vi "AlliGator Load Local IRFs.vi"(8 "error in (no error)":errorcluster, 11 "File Path":path) -> (0 "error out":errorcluster, 1 "Message":string, 2 "IRF Array Time Axis":dbl[](array[numeric]), 3 "[[IRFs]]":dbl[][](array[numeric]), 4 "# IRFs":i32, 5 "Dataset Information v1":T1)   [LabVIEW 2021, in "AlliGator IRF.lvlib"]
uses:
  AlliGator IRF.lvlib
  Files/AlliGator FLI Dataset Information v1.ctl
  <vilib>/addons/h5labview2/file/H5Fmode.ctl
  AlliGator Local IRFs HDF5 File Sections.ctl
  <vilib>/Utility/error.llb/Error Cluster From Error Code.vi
  <vilib>/addons/h5labview2/base/lib_path.vi
  <vilib>/addons/h5labview2/base/H5Equery.vi
  <vilib>/ErrorRing/Error Ring.xnode
  <vilib>/addons/h5labview2/dataset/H5Dread.llb/H5Dread.xnode
  <vilib>/addons/h5labview2/file/H5F.lvlib
  <vilib>/addons/h5labview2/group/H5G.lvlib
  Variant/Variant.lvlib
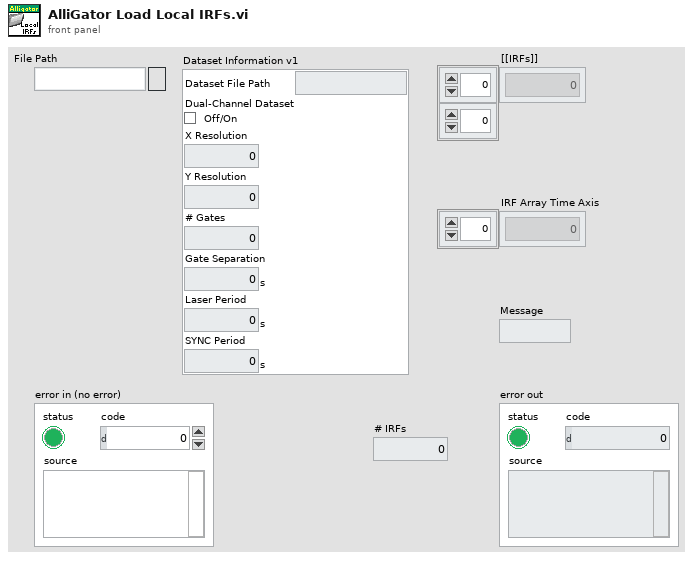
[diagram p1: front panel]
types:
  T1 = typedef "AlliGator IRF.lvlib/AlliGator FLI Dataset Information v1.ctl" = cluster{"Dataset File Path":path, "Dual-Channel Dataset":bool, "X Resolution":i32, "Y Resolution":i32, "# Gates":i32, "Gate Separation":dbl[unit], "Laser Period":dbl[unit], "SYNC Period":dbl[unit]}
  T2 = typedef "AlliGator IRF.lvlib/AlliGator Local IRFs HDF5 File Sections.ctl" = enum16{"File Information", "Dataset Information", "Local IRFs Data"}
  T3 = typedef "H5F.lvlib/H5Fmode.ctl" = enum16{"read-only", "read-write", "overwrite", "create new", "open or create"}
  T4 = typedef "hid_t.ctl" = i64
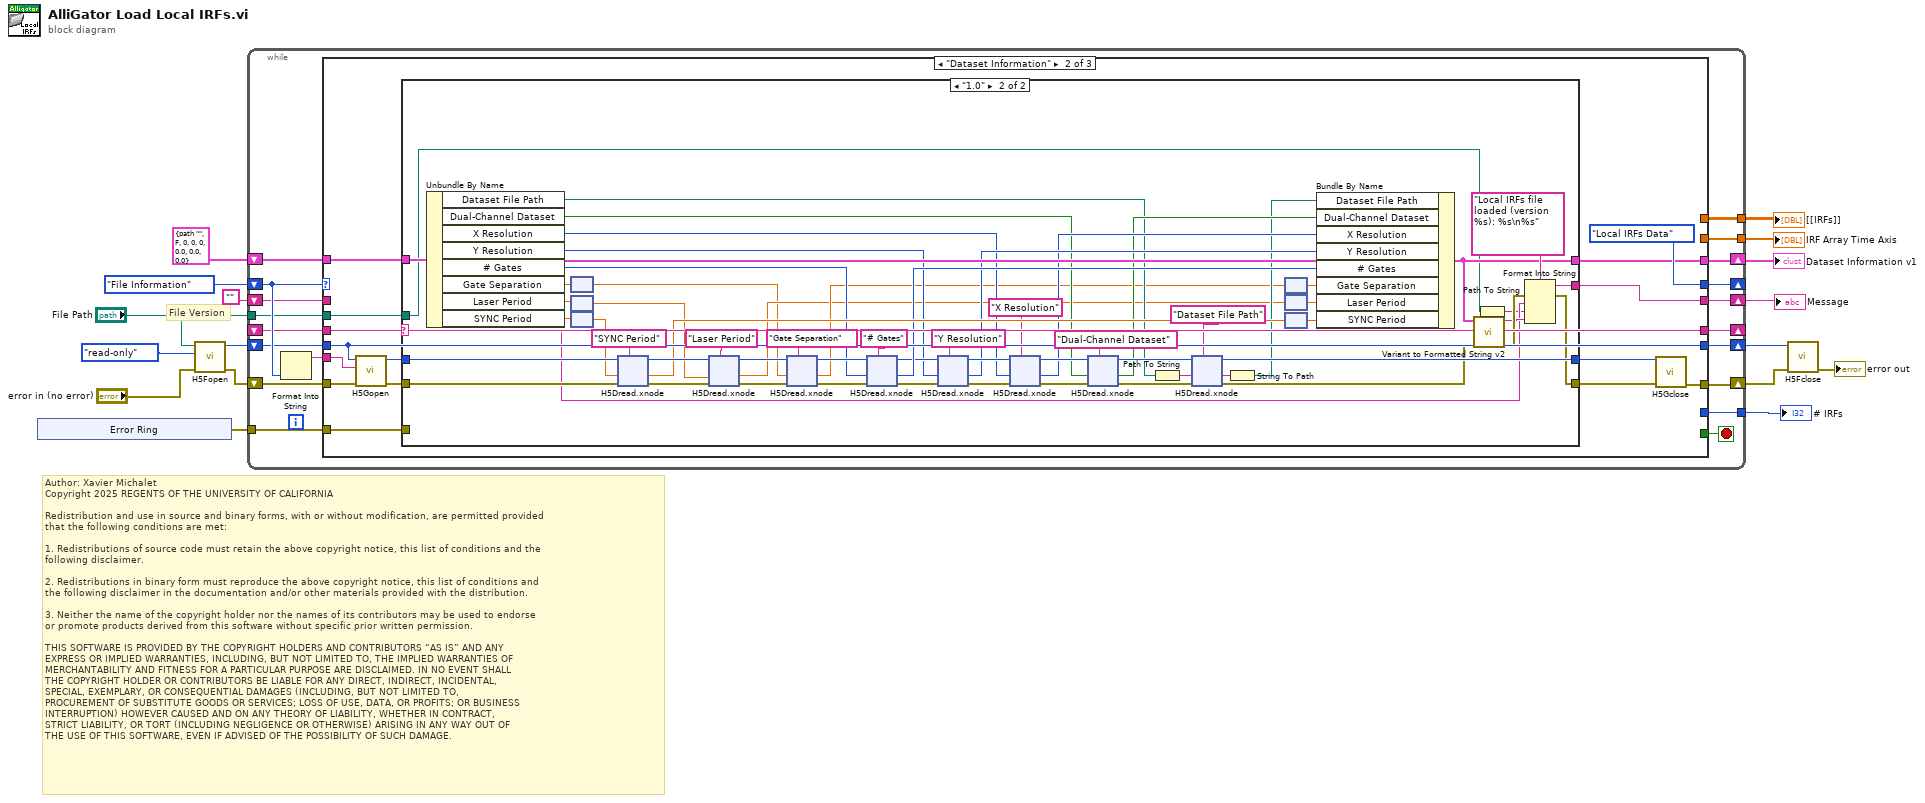
[diagram p0: block diagram]
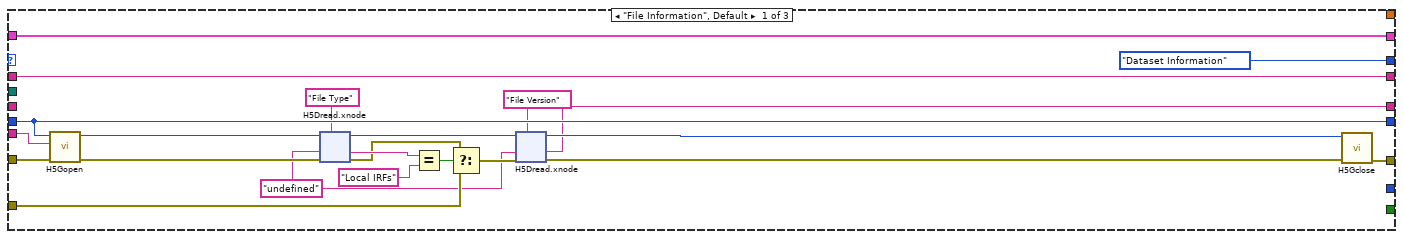
[diagram p2: hidden frame]
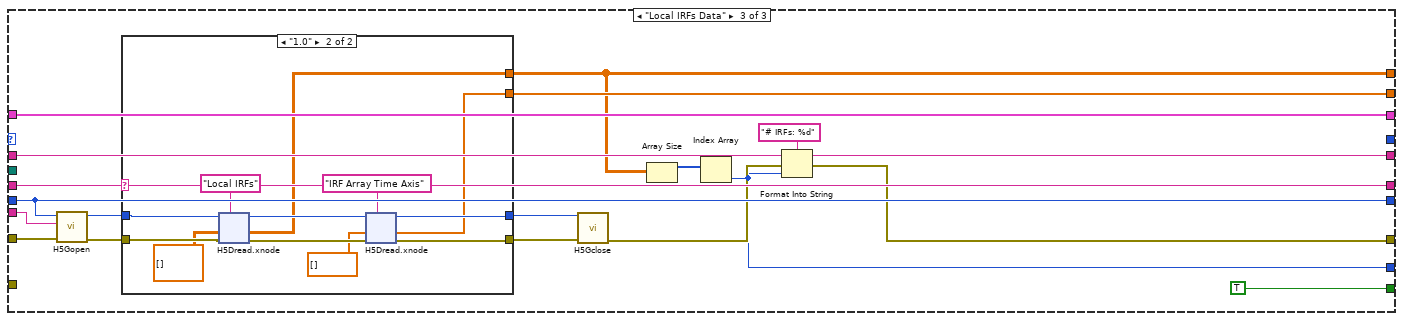
[diagram p4: hidden frame]
diagram:
  # "Author: Xavier Michalet\nCopyright 2025 REGENTS OF THE UNIVERSITY OF CALIFORNIA\n\nRedistribution and use in source and binary forms, with or without modification, are permitted provided\nthat the following conditions are met:\n\n1. Redistributions of source code must retain the above copyright notice, this list of conditions and the\nfollowing disclaimer.\n\n2. Redistributions in binary form must reproduce the above copyright notice, this list of conditions and\nthe following disclaimer in the documentation and/or other materials provided with the distribution.\n\n3. Neither the name of the copyright holder nor the names of its contributors may be used to endorse \nor promote products derived from this software without specific prior written permission.\n\nTHIS SOFTWARE IS PROVIDED BY THE COPYRIGHT HOLDERS AND CONTRIBUTORS “AS IS” AND ANY \nEXPRESS OR IMPLIED WARRANTIES, INCLUDING, BUT NOT LIMITED TO, THE IMPLIED WARRANTIES OF\nMERCHANTABILITY AND FITNESS FOR A PARTICULAR PURPOSE ARE DISCLAIMED. IN NO EVENT SHALL\nTHE COPYRIGHT HOLDER OR CONTRIBUTORS BE LIABLE FOR ANY DIRECT, INDIRECT, INCIDENTAL, \nSPECIAL, EXEMPLARY, OR CONSEQUENTIAL DAMAGES (INCLUDING, BUT NOT LIMITED TO, \nPROCUREMENT OF SUBSTITUTE GOODS OR SERVICES; LOSS OF USE, DATA, OR PROFITS; OR BUSINESS\nINTERRUPTION) HOWEVER CAUSED AND ON ANY THEORY OF LIABILITY, WHETHER IN CONTRACT, \nSTRICT LIABILITY, OR TORT (INCLUDING NEGLIGENCE OR OTHERWISE) ARISING IN ANY WAY OUT OF\nTHE USE OF THIS SOFTWARE, EVEN IF ADVISED OF THE POSSIBILITY OF SUCH DAMAGE."
  # "File Version"
  n1 = xnode "Error Ring"() -> ("error out"=w12:errorcluster)
  n2 = call <vilib>:"H5Fopen.vi"("error in (no error)"="error in (no error)", "mode (read-only)"=H5Fmode."read-only", "path"="File Path") -> ("error out"=w13:errorcluster, "ref out"=w14:T4)  [unwired: 7 in]
  n3 = while {
    shift-right: [w28] -> _
    shift-left: AlliGator_Local_IRFs_HDF5_File_Sections."File Information" -> [w36]
    shift-right: [w33] -> w9
    shift-left: w14 -> [w34]
    shift-right: [w31] -> w8
    shift-left: w13 -> [w32]
    tunnel: w12 -> [w30]
    shift-right: [w29] -> _
    shift-left: _ -> [w27]
    shift-right: [w24] -> w10
    shift-left: T1 {"Dataset File Path"=path "", "Dual-Channel Dataset"=FALSE, "X Resolution"=0, "Y Resolution"=0, "# Gates"=0, "Gate Separation"=0.0, "Laser Period"=0.0, "SYNC Period"=0.0} ("Dataset Information v1") -> [w26]
    shift-right: [w21] -> w4
    shift-left: "" -> [w20]
    tunnel: [w23] -> w7
    tunnel: [w22] -> w6
    tunnel: [w19] -> w3
    tunnel: "File Path" -> [w18]
    stop <- w25 stop-if-true
    n4 = Format Into String(w36) -> (resulting string=w35:string)  [unwired: 3 in, 1 out]
    n5 = case shown="\"Dataset Information\"" w36 {
      tunnel: w35 -> [w57 w102 w294]
      tunnel: w34 -> [w58 w103 w297]
      tunnel: [w58 w103 w297] -> w33
      tunnel: w32 -> [w56 w101 w304]
      tunnel: [w50 w96 w287] -> w31
      tunnel: w30 -> [w44 w95 _]
      tunnel: [w40 w94 w298] -> w29
      tunnel: [AlliGator_Local_IRFs_HDF5_File_Sections."Dataset Information" AlliGator_Local_IRFs_HDF5_File_Sections."Local IRFs Data" _] -> w28
      tunnel: w27 -> [_ w94 w298]
      tunnel: w26 -> [w38 w92 w295]
      tunnel: [_ _ TRUE] -> w25
      tunnel: [w38 w91 w295] -> w24
      tunnel: [_ _ w290] -> w23
      tunnel: [_ _ w296] -> w22
      tunnel: [w37 w90 w291] -> w21
      tunnel: w20 -> [w37 _ w292]
      tunnel: [_ _ w286] -> w19
      tunnel: w18 -> [_ w89 _]
      frame "File Information", Default {
        w42 = "undefined" ("name")
        n6 = call <vilib>:"H5Gopen.vi"("error in (no error)"=w56, "name"=w57, "ref in"=w58) -> ("error out"=w54:errorcluster, "group out"=w55:T4)  [unwired: 7 in]
        n7 = xnode "H5Dread.xnode"("dataset name (this)"="File Type" ("name"), "error in (no error)"=w54, "default"=w42, "ref in"=w55) -> ("error out"=w45:errorcluster, "data"=w48:string, "ref out"=w53:i64)  [unwired: 2 in, 1 out]
        n8 = Equal?(x=w48, y="Local IRFs" ("name")) -> (x = y?=w46:bool)
        n9 = Select(t=w45, s=w46, f=w44) -> (s? t:f=w43:errorcluster)
        n10 = xnode "H5Dread.xnode"("dataset name (this)"="File Version" ("dataset name"), "error in (no error)"=w43, "default"=w42, "ref in"=w53) -> ("error out"=w52:errorcluster, "data"=w40:string, "ref out"=w51:i64)  [unwired: 2 in, 1 out]
        n11 = call <vilib>:"H5Gclose.vi"("error in (no error)"=w52, "group in"=w51) -> ("error out"=w50:errorcluster)  [unwired: 9 in]
      }
      frame "Dataset Information" {
        n12 = call <vilib>:"H5Gopen.vi"("error in (no error)"=w101, "name"=w102, "ref in"=w103) -> ("error out"=w99:errorcluster, "group out"=w100:T4)  [unwired: 7 in]
        n13 = case shown="\"1.0\"" w94 {
          selector: w94 -> [_ w118]
          tunnel: w100 -> [w105 w165]
          tunnel: w99 -> [w104 w164]
          tunnel: [w104 w120] -> w98
          tunnel: [w105 w138] -> w97
          tunnel: w95 -> [_ _]
          tunnel: w92 -> [_ w159]
          tunnel: [_ w123] -> w91
          tunnel: [_ w124] -> w90
          tunnel: w89 -> [_ w107]
          frame "", Default {
          }
          frame "1.0" {
            n14 = Unbundle By Name(w159) -> ("Dataset File Path"=w129:path, "Dual-Channel Dataset"=w131:bool, "X Resolution"=w133:i32, "Y Resolution"=w146:i32, "# Gates"=w151:i32, "Gate Separation"=w111:dbl[unit], "Laser Period"=w110:dbl[unit], "SYNC Period"=w160:dbl[unit])
            n15 = node(w111) -> (w108:dbl)
            n16 = node(w110) -> (w109:dbl)
            n17 = node(w160) -> (w117:dbl)
            n18 = xnode "H5Dread.xnode"("dataset name (this)"="SYNC Period" ("name"), "error in (no error)"=w164, "default"=w117, "ref in"=w165) -> ("error out"=w157:errorcluster, "data"=w158:dbl, "ref out"=w163:i64)  [unwired: 2 in, 1 out]
            n19 = xnode "H5Dread.xnode"("dataset name (this)"="Laser Period" ("dataset name"), "error in (no error)"=w157, "default"=w109, "ref in"=w163) -> ("error out"=w155:errorcluster, "data"=w114:dbl, "ref out"=w156:i64)  [unwired: 2 in, 1 out]
            n20 = xnode "H5Dread.xnode"("dataset name (this)"="Gate Separation" ("dataset name"), "error in (no error)"=w155, "default"=w108, "ref in"=w156) -> ("error out"=w153:errorcluster, "data"=w115:dbl, "ref out"=w154:i64)  [unwired: 2 in, 1 out]
            n21 = xnode "H5Dread.xnode"("dataset name (this)"="# Gates" ("dataset name"), "error in (no error)"=w153, "default"=w151, "ref in"=w154) -> ("error out"=w148:errorcluster, "data"=w149:i32, "ref out"=w147:i64)  [unwired: 2 in, 1 out]
            n22 = xnode "H5Dread.xnode"("dataset name (this)"="Y Resolution" ("dataset name"), "error in (no error)"=w148, "default"=w146, "ref in"=w147) -> ("error out"=w142:errorcluster, "data"=w134:i32, "ref out"=w141:i64)  [unwired: 2 in, 1 out]
            n23 = xnode "H5Dread.xnode"("dataset name (this)"="X Resolution" ("dataset name"), "error in (no error)"=w142, "default"=w133, "ref in"=w141) -> ("error out"=w143:errorcluster, "data"=w132:i32, "ref out"=w140:i64)  [unwired: 2 in, 1 out]
            n24 = xnode "H5Dread.xnode"("dataset name (this)"="Dual-Channel Dataset" ("dataset name"), "error in (no error)"=w143, "default"=w131, "ref in"=w140) -> ("error out"=w144:errorcluster, "data"=w130:bool, "ref out"=w139:i64)  [unwired: 2 in, 1 out]
            n25 = Path To String(path=w129) -> (string=w128:string)
            n26 = xnode "H5Dread.xnode"("dataset name (this)"="Dataset File Path" ("dataset name"), "error in (no error)"=w144, "default"=w128, "ref in"=w139) -> ("error out"=w121:errorcluster, "data"=w125:string, "ref out"=w138:i64)  [unwired: 2 in, 1 out]
            n27 = String To Path(string=w125) -> (path=w127:path)
            n28 = node(w115) -> (w113:dbl[unit])
            n29 = node(w114) -> (w112:dbl[unit])
            n30 = node(w158) -> (w116:dbl[unit])
            n31 = Bundle By Name(cluster=w159, "Dataset File Path"=w127, "Dual-Channel Dataset"=w130, "X Resolution"=w132, "Y Resolution"=w134, "# Gates"=w149, "Gate Separation"=w113, "Laser Period"=w112, "SYNC Period"=w116) -> (w123:T1)
            n32 = call "Variant to Formatted String v2.vi"("error in (no error)"=w121, "Anything"=w123) -> ("error out"=w122:errorcluster, "String"=w119:string)  [unwired: 8 in]
            n33 = Path To String(path=w107) -> (string=w106:string)
            n34 = Format Into String(format string="Local IRFs file loaded (version %s): %s\n%s", error in=w122, w118, w106, w119) -> (resulting string=w124:string, error out=w120:errorcluster)  [unwired: 1 in]
          }
        }
        n35 = call <vilib>:"H5Gclose.vi"("error in (no error)"=w98, "group in"=w97) -> ("error out"=w96:errorcluster)  [unwired: 9 in]
      }
      frame "Local IRFs Data" {
        n36 = call <vilib>:"H5Gopen.vi"("error in (no error)"=w304, "name"=w294, "ref in"=w297) -> ("error out"=w303:errorcluster, "group out"=w302:T4)  [unwired: 7 in]
        n37 = case shown="\"1.0\"" w298 {
          tunnel: w303 -> [w306 w315]
          tunnel: w302 -> [w305 w314]
          tunnel: [w306 w311] -> w301
          tunnel: [w305 w312] -> w300
          tunnel: [_ w309] -> w290
          tunnel: [_ w307] -> w296
          frame "", Default {
          }
          frame "1.0" {
            n38 = xnode "H5Dread.xnode"("dataset name (this)"="Local IRFs" ("name"), "error in (no error)"=w315, "default"=dbl[][] [] ("[[IRFs]]"), "ref in"=w314) -> ("error out"=w318:errorcluster, "data"=w309:dbl[][], "ref out"=w313:i64)  [unwired: 2 in, 1 out]
            n39 = xnode "H5Dread.xnode"("dataset name (this)"="IRF Array Time Axis" ("dataset name"), "error in (no error)"=w318, "default"=dbl[] [] ("IRF Array Time Axis"), "ref in"=w313) -> ("error out"=w311:errorcluster, "data"=w307:dbl[], "ref out"=w312:i64)  [unwired: 2 in, 1 out]
          }
        }
        n40 = call <vilib>:"H5Gclose.vi"("error in (no error)"=w301, "group in"=w300) -> ("error out"=w288:errorcluster)  [unwired: 9 in]
        n41 = Array Size(array=w290) -> (size(s)=w289:i32[])
        n42 = Index Array(array=w289) -> (element=w286:i32)  [unwired: 1 in]
        n43 = Format Into String(format string="# IRFs: %d", initial string=w292, error in=w288, w286) -> (resulting string=w291:string, error out=w287:errorcluster)
      }
    }
  }
  "IRF Array Time Axis" <- w6
  "[[IRFs]]" <- w7
  "Message" <- w4
  "Dataset Information v1" <- w10
  "# IRFs" <- w3
  n44 = call <vilib>:"H5Fclose.vi"("error in (no error)"=w8, "ref"=w9) -> ("error out"=→"error out":errorcluster)  [unwired: 9 in]
